vi "PRAT Macro Get Cycle Time.vi"(8 "Error In":errorcluster, 10 "Seconds Column":i32=1, 11 "Full Cycle Data":string[][](array[string])) -> (0 "Error Out":errorcluster, 3 "Cycle Time (Minutes)":dbl)   [LabVIEW 2016]
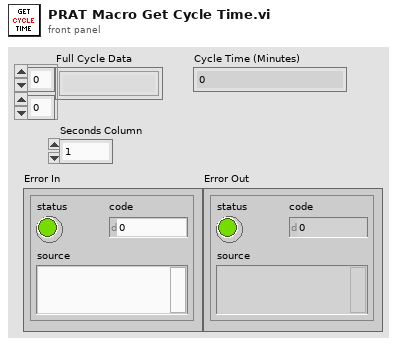
[diagram p1: front panel]
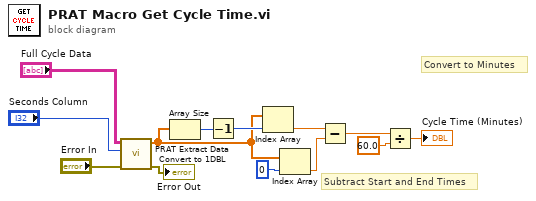
[diagram p0: block diagram]
diagram:
  # "Convert to Minutes"
  # "Subtract Start and End Times"
  n1 = call "PRAT Extract Data Convert to 1DBL.vi"("Error In"="Error In", "Extract Column"="Seconds Column", "Full Cycle Data"="Full Cycle Data") -> ("Error Out"=→"Error Out":errorcluster, "DBL"=w5:dbl[])  [unwired: 7 in]
  n2 = Array Size(array=w5) -> (size(s)=w12:i32)
  n3 = Decrement(x=w12) -> (x-1=w13:i32)
  n4 = Index Array(array=w5, index=w13) -> (element=w7:dbl)
  n5 = Index Array(array=w5, index=0) -> (element=w8:dbl)
  n6 = Subtract(x=w7, y=w8) -> (x-y=w9:dbl)
  n7 = Divide(x=w9, y=60.0) -> (x/y=→"Cycle Time (Minutes)":dbl)
